vi "Create WinMsg Event.vi"(4 "error in (no error)":errorcluster, 5 "Messages (none)":u32[](array[numeric])) -> (0 "error out":errorcluster, 3 "WinMsg Event":refnum<user-event>)   [LabVIEW 2011]
uses:
  Win Msg.ctl
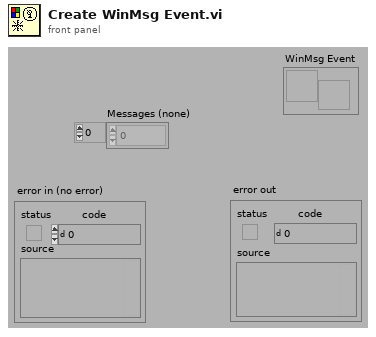
[diagram p1: front panel]
types:
  T1 = typedef "Win Msg.ctl" = cluster{"hWnd":u32, "Msg":u32, "wParam":u32, "lParam":i32, "time":u32, "point":cluster{"X":i32, "Y":i32}}
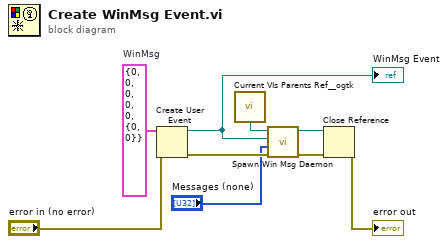
[diagram p0: block diagram]
diagram:
  w9 = T1 {"hWnd"=0, "Msg"=0, "wParam"=0, "lParam"=0, "time"=0, "point"={"X"=0, "Y"=0}}  # WinMsg
  n1 = Create User Event(user event datatype=w9, error in="error in (no error)") -> (user event=w8:refnum<user-event>, error out=w7:errorcluster)
  "WinMsg Event" <- w8
  n2 = call "Current VIs Parents Ref__ogtk.vi"() -> ("Calling VI's Reference"=w5:refnum<vi>)  [unwired: 2 out]
  n3 = call "Spawn Win Msg Daemon.vi"("error in (no error)"=w7, "Messages (none)"="Messages (none)", "WinMsg Event"=w8, "VI Refnum"=w5) -> ("error out"=w3:errorcluster, "dup VI Refnum"=w4:refnum<vi>)  [unwired: 2 out]
  n4 = Close Reference(reference=w4, error in (no error)=w3) -> (error out=→"error out":errorcluster)
